vi "Bitwise Not.vi"(4 "Error":string, 5 "Output Image":T1={"Image ID"=0, "Channel ID"=-1}, 7 "Input Image":T1={"Image ID"=0, "Channel ID"=-1}) -> (0 "Error":string, 1 "Output Image":T1={"Image ID"=0, "Channel ID"=-1}, 3 "Input Image":T1={"Image ID"=0, "Channel ID"=-1})   [LabVIEW 2011, in "labvvis.lvlib"]
doc: "Applies Bitwise NOT to each pixel in Input Image and writes the result to Output Image.\n\nAll images should have the same number of channels. RGBA images are permitted."
uses:
  <userlib>/labvvis/labvvis.lvlib
  <userlib>/labvvis/VVIS Image.ctl
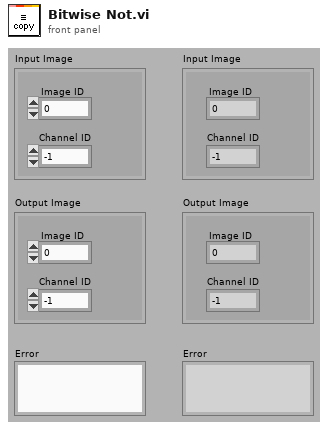
[diagram p1: front panel]
types:
  T1 = typedef "labvvis.lvlib/VVIS Image.ctl" = cluster{"Image ID":i16, "Channel ID":i16}
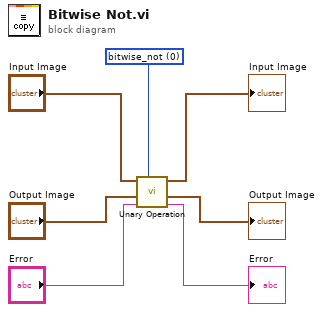
[diagram p0: block diagram]
diagram:
  w1 = u8 0 items=["bitwise_not"] ("Function")
  n1 = call <userlib>:"Unary Operation.vi"("Function"=w1, "Error"="Error", "Output Image"="Output Image", "Input Image"="Input Image") -> ("Error"=→"Error":string, "Output Image"=→"Output Image":T1, "Input Image"=→"Input Image":T1)  [unwired: 2 in]
